vi "Edgertronic-get_caminfo.vi"(3 "error in (no error)":errorcluster, 5 "URL":string="192.168.1.101") -> (0 "error out":errorcluster={"status"=FALSE, "code"=66, "source"="TCP Read in Edgertronic-GET_cmd.vi->Edgertronic-get_caminfo.vi"}, 1 "Cam Info":T1={"Build Date"=timestamp(0 s since 1904-01-01), "Software Build Date"=timestamp(0 s since 1904-01-01), "FPGA Initialized"="1", "Hardware Revision"="6", "Model Number"="1", "Home Dir"="/home/root/ss-web", "IR Filter"="1", "Mac Address"="00:1B:C5:09:61:4D", "Serial Console Enabled"="false", "Serial number"="333", "FPGA Version"="70", "Hardware Configuration"="1", "Connection Information:"="HTTP/1.0 200 OK\r\nContent-Type: text/html; charset=utf-8\r\nContent-Length: 313\r\nConnection: close\r\nDate: Tue, 14 Jun 2016 13:41:45 GMT\r\nServer: lighttpd/1.4.11 (edgertonic slow motion camera)"} {"Software Build Date" format="%<%x>T"; "Build Date" format="%<%x>T"})   [LabVIEW 2015]
doc: "This VI returns all the static camera information."
panel:
  out "data out":string="HTTP/1.0 200 OK\r\nContent-Type: text/html; charset=utf-8\r\nContent-Length: 313\r\nConnection: close\r\nDate: Tue, 14 Jun 2016 13:41:45 GMT\r\nServer: lighttpd/1.4.11 (edgertonic slow motion camera)\r\n\r\n{\"build_date\": \"20150112\", \"sw_build_date\": \"20140911165611\", \"fpga_initialized\": 1, \"hardware_revision\": 6, \"model_number\": 1, \"home_dir\": \"/home/root/ss-web\", \"ir_filter\": 1, \"mac_addr\": \"00:1B:C5:09:61:4D\", \"serial_console_enabled\": false, \"serial_number\": 333, \"fpga_version\": 70, \"hardware_configuration\": 1}"
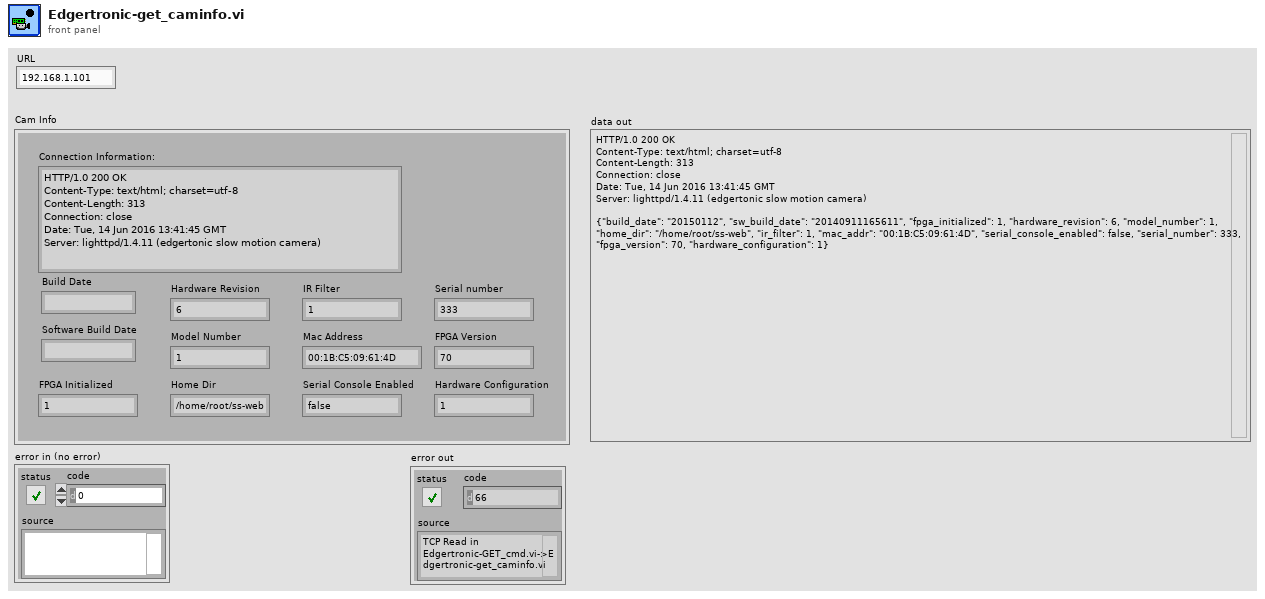
[diagram p1: front panel]
types:
  T1 = cluster{"Build Date":timestamp, "Software Build Date":timestamp, "FPGA Initialized":string, "Hardware Revision":string, "Model Number":string, "Home Dir":string, "IR Filter":string, "Mac Address":string, "Serial Console Enabled":string, "Serial number":string, "FPGA Version":string, "Hardware Configuration":string, "Connection Information:":string}
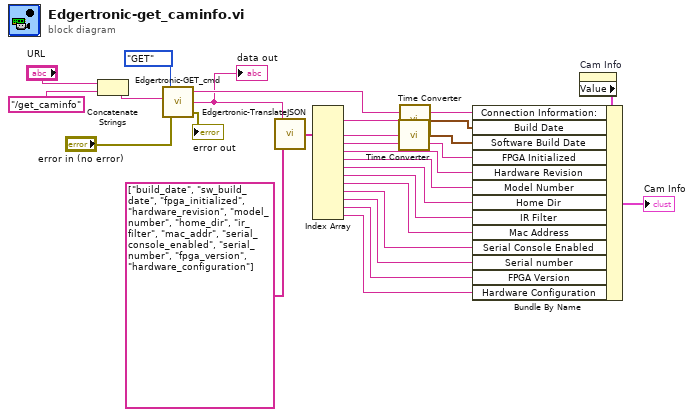
[diagram p0: block diagram]
diagram:
  n1 = Concatenate Strings("URL", "/get_caminfo" ("GET Cmd")) -> (w2:string)
  n2 = call "Edgertronic-GET_cmd.vi"("error in (no error)"="error in (no error)", "URL"=w2, "Type"=enum16{"GET", "POST"}."GET") -> ("error out"=→"error out":errorcluster, "data"=w1:string, "Connection Info"=w23:string)  [unwired: 1 in]
  "data out" <- w1
  n3 = call "Edgertronic-TranslateJSON.vi"("Commands"=string[] ["build_date", "sw_build_date", "fpga_initialized", "hardware_revision", "model_number", "home_dir", "ir_filter", "mac_addr", "serial_console_enabled", "serial_number", "fpga_version", "hardware_configuration"], "data"=w1) -> ("Values"=w22:string[])  [unwired: 3 in]
  n4 = Index Array(array=w22) -> (element #1=w10:string, element #2=w8:string, element #3=w21:string, element #4=w20:string, element #5=w19:string, element #6=w18:string, element #7=w17:string, element #8=w16:string, element #9=w15:string, element #10=w14:string, element #11=w13:string, element #12=w12:string)  [unwired: 12 in]
  n5 = call "Time Converter.vi"("data"=w8) -> ("time stamp"=w7:timestamp)
  n6 = call "Time Converter.vi"("data"=w10) -> ("time stamp"=w9:timestamp)
  n7 = property on="Cam Info" class="Clust (strict)"() -> ("Value"=w24:T1)  [unwired: 2 in, 2 out]
  n8 = Bundle By Name(cluster=w24, "Connection Information:"=w23, "Build Date"=w9, "Software Build Date"=w7, "FPGA Initialized"=w21, "Hardware Revision"=w20, "Model Number"=w19, "Home Dir"=w18, "IR Filter"=w17, "Mac Address"=w16, "Serial Console Enabled"=w15, "Serial number"=w14, "FPGA Version"=w13, "Hardware Configuration"=w12) -> (→"Cam Info":T1)
